vi "component center offset.vi"() -> ()   [LabVIEW 2018]
uses:
  <vilib>/Analysis/NI_AALPro.lvlib
  <vilib>/Analysis/coordinate.llb/2D Cartesian Coordinate Rotation (Scalar).vi
panel:
  out "Numeric":dbl
  out "BP rotation":dbl
  out "XY offset":dbl[](array[numeric])
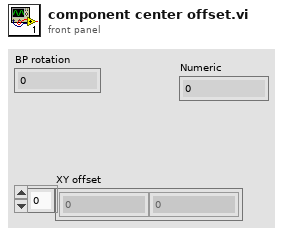
[diagram p1: front panel]
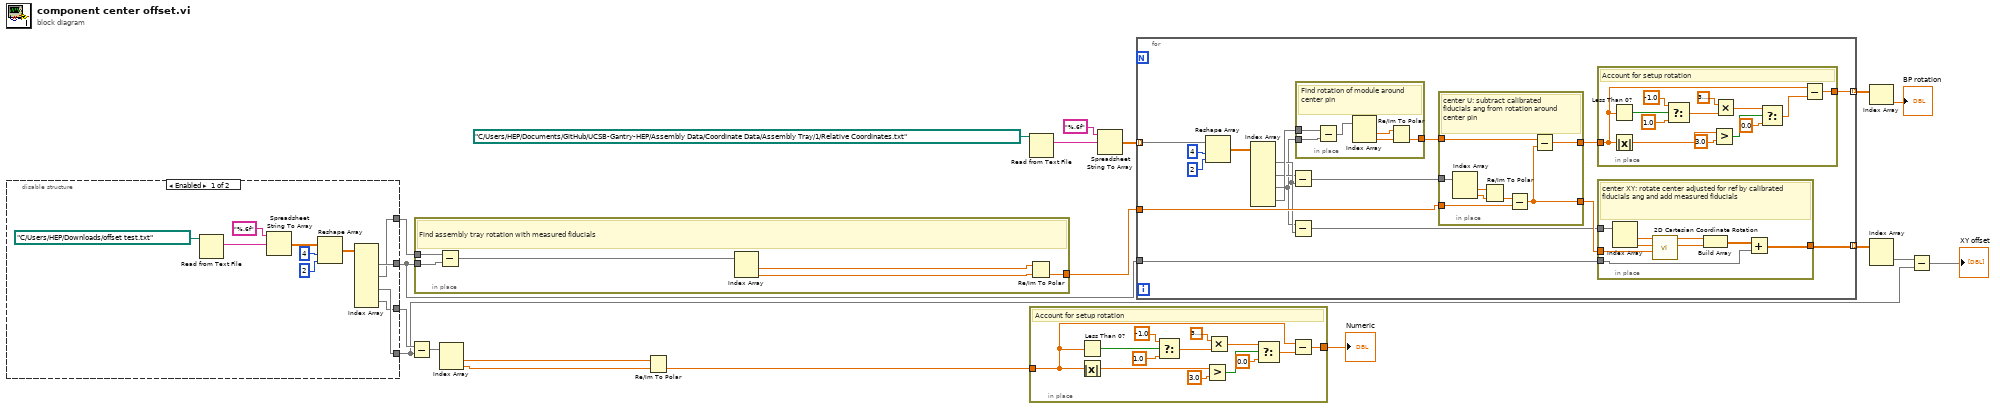
[diagram p0: block diagram]
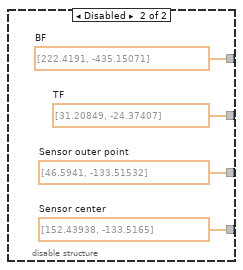
[diagram p2: hidden frame]
diagram:
  n1 = disable-structure shown="Enabled" {
    disable-tunnel: [w22 w34] -> w6
    disable-tunnel: [w23 w32] -> w11
    disable-tunnel: [w24 w33] -> w10
    disable-tunnel: [w21 w31] -> w7
    frame Enabled {
      n2 = Read from Text File(file (use dialog)=path "C:/Users/HEP/Downloads/offset test.txt") -> (text=w30:string)  [unwired: 3 in, 3 out]
      n3 = Spreadsheet String To Array(format string="%.6f", spreadsheet string=w30) -> (array=w28:dbl[][])  [unwired: 2 in]
      n4 = Reshape Array(w28, 4 ("dimension size"), 2 ("dimension size")) -> (w27:dbl[][])
      n5 = Index Array(array=w27) -> (element #1=w24:dbl[], element #2=w23:dbl[], element #3=w22:dbl[], element #4=w21:dbl[])  [unwired: 8 in]
    }
    frame Disabled {
      w31 = dbl[] [46.5941, -133.51532]  # Sensor outer point
      w32 = dbl[] [222.4191, -435.15071]  # BF
      w33 = dbl[] [31.20849, -24.37407]  # TF
      w34 = dbl[] [152.43938, -133.5165]  # Sensor center
    }
  }
  n6 = Subtract(x=w7, y=w6) -> (x-y=w5:dbl[])
  n7 = in-place {
    in-place-border: [w38] -> w16
    in-place-border: w11 -> [w36]
    in-place-border: w10 -> [w35]
    # "Find assembly tray rotation with measured fiducials"
    n8 = Subtract(x=w36, y=w35) -> (x-y=w37:dbl[])
    n9 = Index Array(array=w37) -> (element #1=w39:dbl, element #2=w40:dbl)  [unwired: 2 in]
    n10 = Re/Im To Polar(2:w40, 3:w39) -> (0:w38:dbl)  [unwired: 1 out]
  }
  n11 = Index Array(array=w5) -> (element #1=w4:dbl, element #2=w3:dbl)  [unwired: 2 in]
  n12 = Re/Im To Polar(2:w3, 3:w4) -> (0:w2:dbl)  [unwired: 1 out]
  n13 = Read from Text File(file (use dialog)=path "C:/Users/HEP/Documents/GitHub/UCSB-Gantry-HEP/Assembly Data/Coordinate Data/Assembly Tray/1/Relative Coordinates.txt") -> (text=w19:string)  [unwired: 3 in, 3 out]
  n14 = in-place {
    in-place-border: [w42] -> w1
    in-place-border: w2 -> [w41]
    # "Account for setup rotation"
    n15 = Less Than 0?(x=w41) -> (x < 0?=w53:bool)
    n16 = Absolute Value(x=w41) -> (abs(x)=w50:dbl)
    n17 = Select(t=-1.0, s=w53, f=1.0) -> (s? t:f=w44:dbl)
    n18 = Greater?(x=w50, y=3.0) -> (0:w48:bool)
    n19 = Multiply(x=3.141592653589793, y=w44) -> (x*y=w43:dbl)
    n20 = Select(t=w43, s=w48, f=0.0) -> (s? t:f=w46:dbl)
    n21 = Subtract(x=w41, y=w46) -> (x-y=w42:dbl)
  }
  "Numeric" <- w1
  n22 = Spreadsheet String To Array(format string="%.6f", spreadsheet string=w19) -> (array=w15:dbl[][])  [unwired: 2 in]
  n23 = for {
    tunnel: w15 -> [w66] mode=indexing
    tunnel: w10 -> [w68]
    tunnel: w16 -> [w67]
    tunnel: [w56] -> w14 mode=indexing
    tunnel: [w54] -> w9 mode=indexing
    n24 = Reshape Array(w66, 4 ("dimension size"), 2 ("dimension size")) -> (w63:dbl[][])
    n25 = Index Array(array=w63) -> (element #1=w61:dbl[], element #2=w60:dbl[], element #3=w59:dbl[], element #4=w62:dbl[])  [unwired: 8 in]
    n26 = Subtract(x=w60, y=w61) -> (x-y=w57:dbl[])
    n27 = Subtract(x=w59, y=w61) -> (x-y=w58:dbl[])
    n28 = in-place {
      in-place-border: [w89] -> w70
      in-place-border: w62 -> [w88]
      in-place-border: w59 -> [w84]
      # "Find rotation of module around center pin"
      n29 = Subtract(x=w88, y=w84) -> (x-y=w87:dbl[])
      n30 = Index Array(array=w87) -> (element #1=w86:dbl, element #2=w85:dbl)  [unwired: 2 in]
      n31 = Re/Im To Polar(2:w85, 3:w86) -> (0:w89:dbl)  [unwired: 1 out]
    }
    n32 = in-place {
      in-place-border: w70 -> [w96]
      in-place-border: [w90] -> w69
      in-place-border: w67 -> [w95]
      in-place-border: [w93] -> w55
      in-place-border: w57 -> [w92]
      # "center U: subtract calibrated fiducials ang from rotation around center pin"
      n33 = Index Array ("ref BF - TF")(array=w92) -> (element #1=w94:dbl, element #2=w97:dbl)  [unwired: 2 in]
      n34 = Re/Im To Polar(2:w97, 3:w94) -> (0:w91:dbl)  [unwired: 1 out]
      n35 = Subtract ("fiducials ref - measured")(x=w91, y=w95) -> (x-y=w90:dbl)
      n36 = Subtract ("center to outer ang - (ref - measured)")(x=w96, y=w90) -> (x-y=w93:dbl)
    }
    n37 = in-place {
      in-place-border: [w72] -> w54
      in-place-border: w55 -> [w71]
      # "Account for setup rotation"
      n38 = Less Than 0?(x=w71) -> (x < 0?=w83:bool)
      n39 = Absolute Value(x=w71) -> (abs(x)=w80:dbl)
      n40 = Select(t=-1.0, s=w83, f=1.0) -> (s? t:f=w74:dbl)
      n41 = Greater?(x=w80, y=3.0) -> (0:w78:bool)
      n42 = Multiply(x=3.141592653589793, y=w74) -> (x*y=w73:dbl)
      n43 = Select(t=w73, s=w78, f=0.0) -> (s? t:f=w76:dbl)
      n44 = Subtract(x=w71, y=w76) -> (x-y=w72:dbl)
    }
    n45 = in-place {
      in-place-border: [w101] -> w56
      in-place-border: w69 -> [w100]
      in-place-border: w68 -> [w99]
      in-place-border: w58 -> [w98]
      # "center XY: rotate center adjusted for ref by calibrated fiducials ang and add measured fiducials"
      n46 = Index Array ("center pin - TF ref")(array=w98) -> (element #1=w106:dbl, element #2=w105:dbl)  [unwired: 2 in]
      n47 = call-poly <vilib>:"2D Cartesian Coordinate Rotation.vi"("theta"=w100, "y"=w105, "x"=w106) -> ("y out"=w102:dbl, "x out"=w103:dbl)  [unwired: 6 in, 1 out]
      n48 = Build Array ("rotated XY for center pin")(w103, w102) -> (w104:dbl[])
      n49 = Add ("fit onto measured fiducials")(x=w104, y=w99) -> (x+y=w101:dbl[])
    }
  }
  n50 = Index Array(array=w9) -> (element=→"BP rotation":dbl)  [unwired: 1 in]
  n51 = Index Array(array=w14) -> (element=w13:dbl[])  [unwired: 2 in]
  n52 = Subtract(x=w13, y=w6) -> (x-y=→"XY offset":dbl[])
